vi "Create DataBindings.vi"(8 "error in (no error)":errorcluster caption="错误输入（无错误）", 9 "DataMember":string, 10 "DataGridView":refnum<k24>, 11 "OleDBClass 输入":refnum<class "OleDBClass.lvclass"> caption="DNL_LabVIEW Object in") -> (0 "error out":errorcluster caption="错误输出", 3 "OleDBClass 输出":refnum<class "OleDBClass.lvclass"> caption="DNL_LabVIEW Object out")   [LabVIEW 2012, in "OleDBClass.lvclass"]
uses:
  OleDBClass.lvclass
  System.Windows.Forms
  OleDBClass.lvclass/OleDBClass.ctl
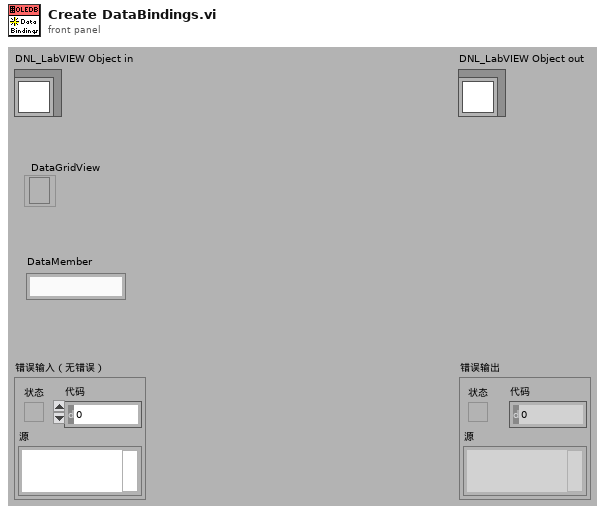
[diagram p1: front panel]
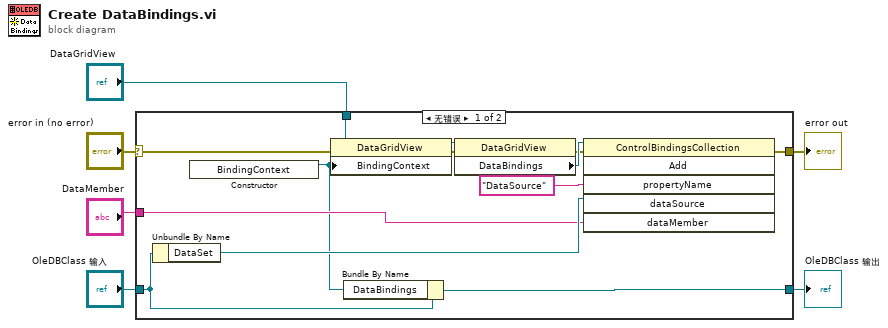
[diagram p0: block diagram]
diagram:
  n1 = case shown="无错误" "error in (no error)" {
    selector: "error in (no error)" -> [w7 w21]
    tunnel: [w8 w21] -> w5
    tunnel: [w9 w20] -> w3
    tunnel: "OleDBClass 输入" -> [w11 w20]
    tunnel: "DataGridView" -> [w19 _]
    tunnel: "DataMember" -> [w12 _]
    frame No Error {
      n2 = Unbundle By Name(w11) -> ("DataSet"=w14:refnum<k24>)
      n3 = constructor class="BindingContext"() -> (reference out=w10:refnum<k24>)  [unwired: 3 in, 2 out]
      n4 = property class="DataGridView"(reference=w19, error in=w7, "BindingContext"=w10) -> (reference out=w18:refnum<k24>, error out=w17:errorcluster)
      n5 = Bundle By Name(cluster=w11, "DataBindings"=w10) -> (w9:refnum<class "OleDBClass.lvclass">)
      n6 = property class="DataGridView"(reference=w18, error in=w17) -> (error out=w15:errorcluster, "DataBindings"=w16:refnum<k24>)  [unwired: 1 out]
      n7 = invoke class="ControlBindingsCollection" method="Add"(reference=w16, error in=w15, "propertyName"="DataSource", "dataSource"=w14, "dataMember"=w12) -> (error out=w8:errorcluster)  [unwired: 1 in, 5 out]
    }
    frame Error {
    }
  }
  "error out" <- w5
  "OleDBClass 输出" <- w3
